vi "temperature control notification.vi"() -> ()   [LabVIEW 2018]
panel:
  out "Boolean":bool
  out "String":string
  in  "Numeric":dbl
  out "Thermometer":dbl(slide) scale=0.0..100.0
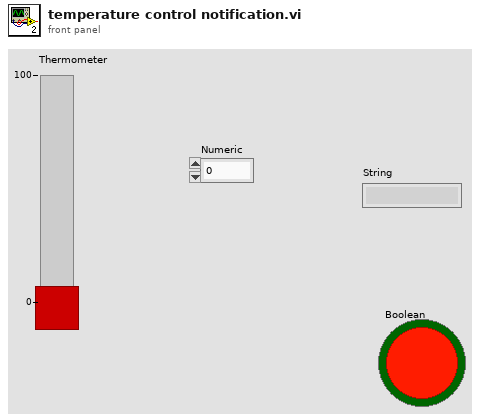
[diagram p1: front panel]
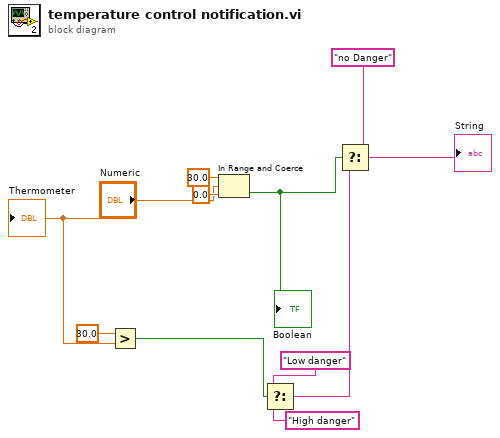
[diagram p0: block diagram]
diagram:
  n1 = Greater?(x=30.0, y="Numeric") -> (0:w4:bool)
  n2 = In Range and Coerce(upper limit=30.0, x="Numeric", lower limit=0.0) -> (In Range?=w7:bool)  [unwired: 1 out]
  "Boolean" <- w7
  n3 = Select(t="Low danger", s=w4, f="High danger") -> (s? t:f=w1:string)
  n4 = Select(t="no Danger", s=w7, f=w1) -> (s? t:f=→"String":string)
  "Thermometer" <- "Numeric"
